vi "WLAN ModAcc Fetch.vi"(0 "Instrument Handle In":refnum<k21>, 1 "Selector String":string, 11 "error in (no error)":errorcluster) -> (4 "Instrument Handle Out":refnum<k21>, 6 "WLAN ModAcc Results":T1 {"Composite Pilot RMS EVM Mean (dB)" format="%.2f"; "Composite Data RMS EVM Mean (dB)" format="%.2f"; "Composite RMS EVM Mean (dB)" format="%.2f"}, 15 "error out":errorcluster)   [LabVIEW 2018, in "RFmxWLAN.lvlib"]
uses:
  RFmxWLAN.lvlib
  Typedefs/WLAN ModAcc Results.ctl
  <vilib>/RFmx/WLAN/mx/RFmxWLAN.llb/RFmxWLAN OFDMModAcc Fetch Chain RMS EVM per Symbol Mean Trace.vi
  <vilib>/RFmx/WLAN/mx/RFmxWLAN.llb/RFmxWLAN OFDMModAcc Fetch Data Constellation Trace.vi
  <vilib>/RFmx/WLAN/mx/RFmxWLAN.llb/RFmxWLAN OFDMModAcc Fetch Composite RMS EVM.vi
  <vilib>/RFmx/WLAN/mx/RFmxWLAN.llb/RFmxWLAN OFDMModAcc Fetch Number of Symbols Used.vi
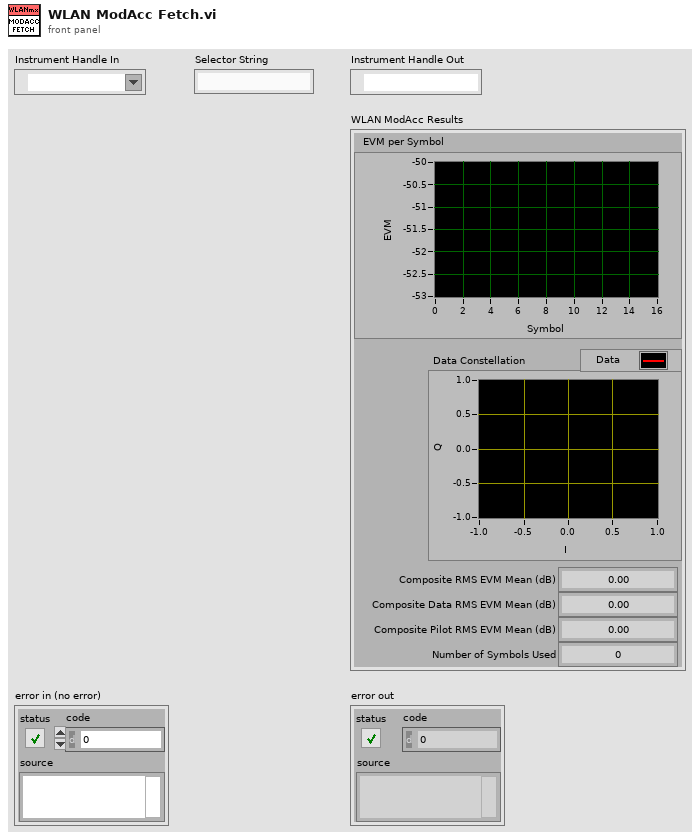
[diagram p1: front panel]
types:
  T1 = typedef "RFmxWLAN.lvlib/WLAN ModAcc Results.ctl" = cluster{"EVM per Symbol":cluster{"x0":dbl, "dx":dbl, "y":sgl[]}, "Data Constellation":csg[], "Composite RMS EVM Mean (dB)":dbl, "Composite Data RMS EVM Mean (dB)":dbl, "Composite Pilot RMS EVM Mean (dB)":dbl, "Number of Symbols Used":i32}
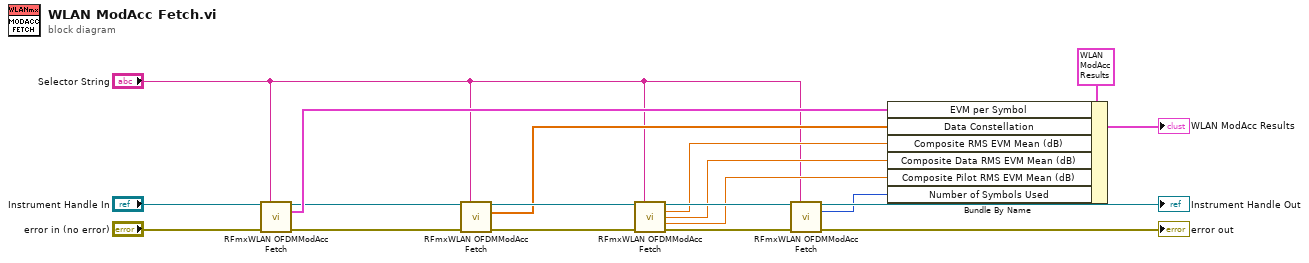
[diagram p0: block diagram]
diagram:
  n1 = call-poly <vilib>:"RFmxWLAN OFDMModAcc Fetch.vi"("Instrument Handle In"="Instrument Handle In", "Selector String"="Selector String", "error in (no error)"="error in (no error)") -> ("Instrument Handle Out"=w4:refnum<k21>, "Chain RMS EVM per Symbol Mean (dB or %)"=w11:cluster{"x0":dbl, "dx":dbl, "y":sgl[]}, "error out"=w19:errorcluster)  [unwired: 10 in]
  n2 = call-poly <vilib>:"RFmxWLAN OFDMModAcc Fetch.vi"("Instrument Handle In"=w4, "Selector String"="Selector String", "error in (no error)"=w19) -> ("Instrument Handle Out"=w3:refnum<k21>, "Data Constellation"=w2:csg[], "error out"=w5:errorcluster)  [unwired: 10 in]
  n3 = call-poly <vilib>:"RFmxWLAN OFDMModAcc Fetch.vi"("Instrument Handle In"=w3, "Selector String"="Selector String", "error in (no error)"=w5) -> ("Instrument Handle Out"=w13:refnum<k21>, "Composite RMS EVM Mean (dB or %)"=w9:dbl, "Composite Data RMS EVM Mean (dB or %)"=w8:dbl, "Composite Pilot RMS EVM Mean (dB or %)"=w7:dbl, "error out"=w18:errorcluster)  [unwired: 8 in]
  n4 = call-poly <vilib>:"RFmxWLAN OFDMModAcc Fetch.vi"("Instrument Handle In"=w13, "Selector String"="Selector String", "error in (no error)"=w18) -> ("Instrument Handle Out"=→"Instrument Handle Out":refnum<k21>, "Number of Symbols Used"=w6:i32, "error out"=→"error out":errorcluster)  [unwired: 10 in]
  n5 = Bundle By Name(cluster=T1 {"EVM per Symbol"={"x0"=0.0, "dx"=0.0, "y"=[]}, "Data Constellation"=[], "Composite RMS EVM Mean (dB)"=0.0, "Composite Data RMS EVM Mean (dB)"=0.0, "Composite Pilot RMS EVM Mean (dB)"=0.0, "Number of Symbols Used"=0} ("WLAN ModAcc Results"), "EVM per Symbol"=w11, "Data Constellation"=w2, "Composite RMS EVM Mean (dB)"=w9, "Composite Data RMS EVM Mean (dB)"=w8, "Composite Pilot RMS EVM Mean (dB)"=w7, "Number of Symbols Used"=w6) -> (→"WLAN ModAcc Results":T1)
